vi "DSF.Transceiver.GE Reflective Memory.Set VISA Resource Name.vi"(10 "VISA resource name":refnum<visa-resource-name>, 11 "GE Reflective Memory in":refnum<class "DSF.Transceiver.GE Reflective Memory.lvclass">) -> (3 "GE Reflective Memory out":refnum<class "DSF.Transceiver.GE Reflective Memory.lvclass">)   [LabVIEW 2017, in "DSF.Transceiver.GE Reflective Memory.lvlib" / "DSF.Transceiver.GE Reflective Memory.lvclass"]
uses:
  DSF.Transceiver.GE Reflective Memory.lvclass
  DSF.Transceiver.GE Reflective Memory.lvclass/DSF.Transceiver.GE Reflective Memory.ctl
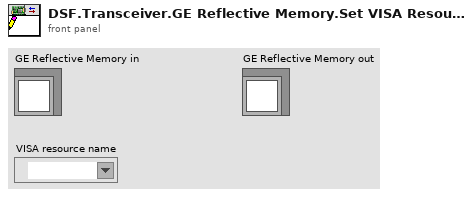
[diagram p1: front panel]
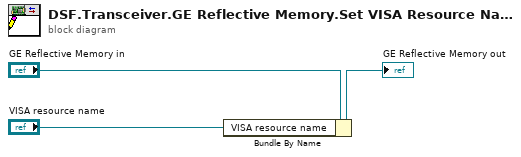
[diagram p0: block diagram]
diagram:
  n1 = Bundle By Name(cluster="GE Reflective Memory in", "VISA resource name"="VISA resource name") -> (→"GE Reflective Memory out":refnum<class "DSF.Transceiver.GE Reflective Memory.lvclass">)
